vi "Build_Asylum_ReadValue.vi"(8 "error in (no error)":errorcluster, 11 "Value":string) -> (0 "error out":errorcluster, 3 "String":string)   [LabVIEW 2019]
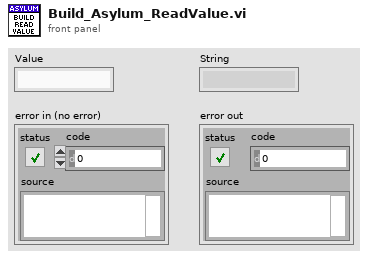
[diagram p1: front panel]
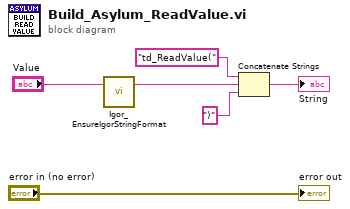
[diagram p0: block diagram]
diagram:
  n1 = call "Igor_EnsureIgorStringFormat.vi"("Value"="Value") -> ("Value"=w5:string)  [unwired: 2 in]
  n2 = Concatenate Strings("td_ReadValue(", w5, ")" ("y")) -> (→"String":string)
  "error out" <- "error in (no error)"
